vi "Read Label.vi"(8 "error in (no error)":errorcluster, 10 "Label":string, 11 "gScript Interpreter in":refnum<class "gScript Interpreter.lvclass">) -> (0 "error out":errorcluster, 1 "Arguments":string[](array[string]), 2 "Line":i32, 3 "gScript Interpreter out":refnum<class "gScript Interpreter.lvclass">)   [LabVIEW 2017, in "gScript Interpreter.lvclass"]
uses:
  gScript Interpreter.lvclass
  gScript Interpreter.lvclass/gScript Interpreter.ctl
  <vilib>/Utility/error.llb/Error Cluster From Error Code.vi
  <vilib>/ErrorRing/Error Ring.xnode
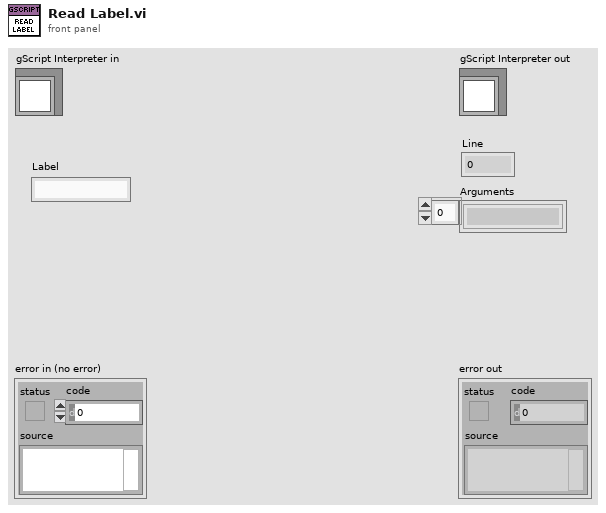
[diagram p1: front panel]
types:
  T1 = typedef "Label.ctl" = cluster{"Label":string, "Line":i32, "Arguments":string[]}
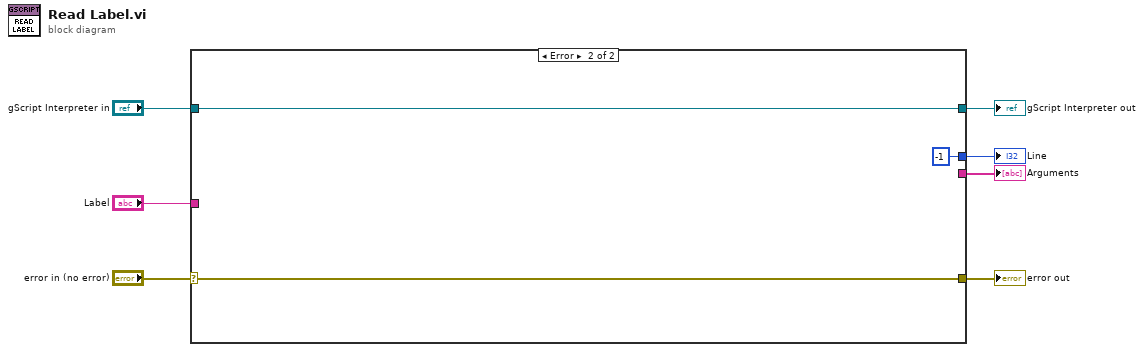
[diagram p0: block diagram]
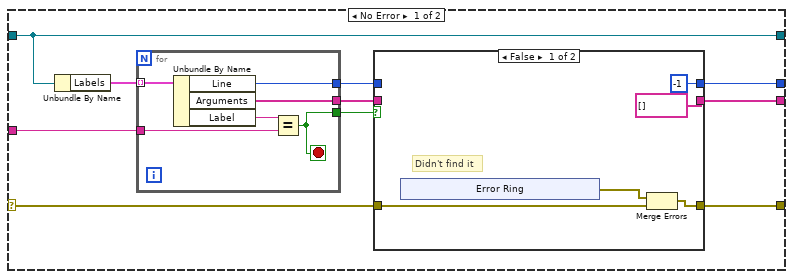
[diagram p2: hidden frame]
diagram:
  n1 = case shown="Error" "error in (no error)" {
    selector: "error in (no error)" -> [w11 w38]
    tunnel: [w10 w38] -> w6
    tunnel: [w17 w37] -> w4
    tunnel: "gScript Interpreter in" -> [w17 w37]
    tunnel: "Label" -> [w15 _]
    tunnel: [w12 -1 ("Line")] -> w2
    tunnel: [w8 _] -> w1
    frame No Error {
      n2 = Unbundle By Name(w17) -> ("Labels"=w16:T1[])
      n3 = for {
        tunnel: w16 -> [w35] mode=indexing
        tunnel: w15 -> [w34]
        tunnel: [w33] -> w13
        tunnel: [w32] -> w14
        tunnel: [w30] -> w9
        stop <- w32 stop-if-true
        n4 = Unbundle By Name(w35) -> ("Line"=w33:i32, "Arguments"=w30:string[], "Label"=w31:string)
        n5 = Equal?(x=w31, y=w34) -> (x = y?=w32:bool)
      }
      n6 = case shown="False" w14 {
        tunnel: w13 -> [_ w29]
        tunnel: [-1 ("Line") w29] -> w12
        tunnel: w11 -> [w21 w28]
        tunnel: [w20 w28] -> w10
        tunnel: w9 -> [_ w27]
        tunnel: [string[] [] ("Arguments") w27] -> w8
        frame False {
          # "Didn't find it"
          n7 = xnode "Error Ring"() -> ("error out"=w22:errorcluster)
          n8 = Merge Errors(w22, w21) -> (w20:errorcluster)
        }
        frame True {
          # "Found it"
        }
      }
    }
    frame Error {
    }
  }
  "error out" <- w6
  "gScript Interpreter out" <- w4
  "Line" <- w2
  "Arguments" <- w1
